vi "Enable Disable Comparator.vi"(7 "Disable?":bool=TRUE, 8 "error in (no error)":errorcluster, 10 "Tree":string, 11 "TreeControl in":refnum<vi>) -> (0 "error out":errorcluster)   [LabVIEW 2018, in "Test Manager.lvlib"]
uses:
  Test Manager.lvlib
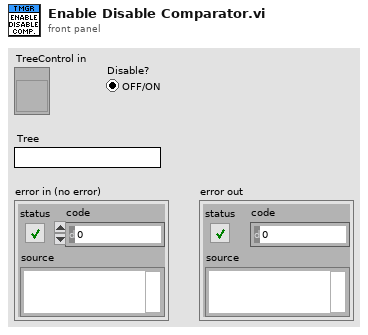
[diagram p1: front panel]
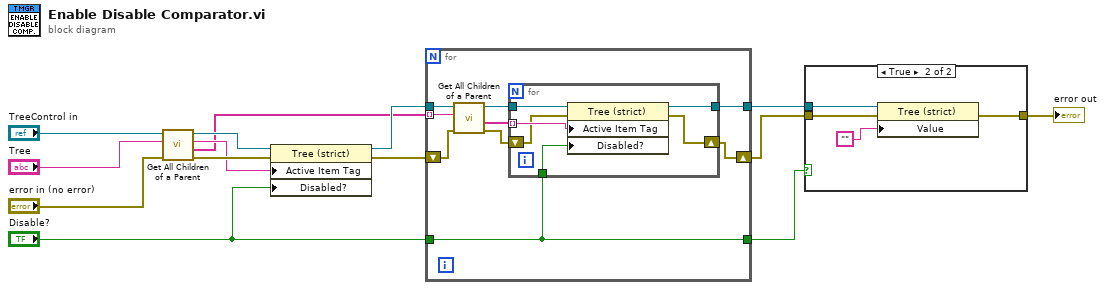
[diagram p0: block diagram]
diagram:
  n1 = call "Get All Children of a Parent.vi"("Error In"="error in (no error)", "Parent tag"="Tree", "Tree ref"="TreeControl in") -> ("Error out"=w13:errorcluster, "All Children"=w8:string[], "Parent tag out"=w11:string, "Tree ref out"=w9:refnum<vi>)  [unwired: 5 in]
  n2 = property class="Tree (strict)"(reference=w9, error in=w13, "Active Item Tag"=w11, "Disabled?"="Disable?") -> (reference out=w10:refnum<vi>, error out=w14:errorcluster)
  n3 = for {
    tunnel: w10 -> [w21]
    tunnel: w8 -> [w23] mode=indexing
    shift-right: [w18] -> w3
    shift-left: w14 -> [w19]
    tunnel: "Disable?" -> [w15]
    tunnel: [w16] -> w4
    tunnel: [w15] -> w1
    n4 = call "Get All Children of a Parent.vi"("Error In"=w19, "Parent tag"=w23, "Tree ref"=w21) -> ("Error out"=w17:errorcluster, "All Children"=w20:string[], "Tree ref out"=w22:refnum<vi>)  [unwired: 5 in, 1 out]
    n5 = for {
      tunnel: w22 -> [w29]
      tunnel: w20 -> [w28] mode=indexing
      shift-right: [w27] -> w18
      shift-left: w17 -> [w26]
      tunnel: w15 -> [w25]
      tunnel: [w24] -> w16
      n6 = property class="Tree (strict)"(reference=w29, error in=w26, "Active Item Tag"=w28, "Disabled?"=w25) -> (reference out=w24:refnum<vi>, error out=w27:errorcluster)
    }
  }
  n7 = case shown="True" w1 {
    tunnel: w4 -> [_ w34]
    tunnel: w3 -> [w30 w33]
    tunnel: [w30 w31] -> w2
    frame False {
    }
    frame True {
      n8 = property class="Tree (strict)"(reference=w34, error in=w33, "Value"="") -> (error out=w31:errorcluster)  [unwired: 1 out]
    }
  }
  "error out" <- w2
